vi "Server Fix.vi"() -> ()   [LabVIEW 2017]
uses:
  <vilib>/Analysis/Matrix/Datatypes/RealMatrix.ctl
  <vilib>/Platform/TimedLoop/XDataNode/timing_clust.ctl
  <vilib>/Platform/TimedLoop/XDataNode/nitl_modes.ctl
  <vilib>/Platform/TimedLoop/XDataNode/wakeup.ctl
  <vilib>/platform/TimedLoop/XDataNode/XDataNode.xnode
  <vilib>/Platform/TimedLoop/XDataNode/XDNodeRunTimeDep.lvlib
  <vilib>/Analysis/Matrix/NI_Matrix.lvlib
panel:
  in  "Processor":i32=-2
  out "?":string="SERVER"
  out "BYTE WRITE FROM SERVER":i32
  in  "Matrix":T1
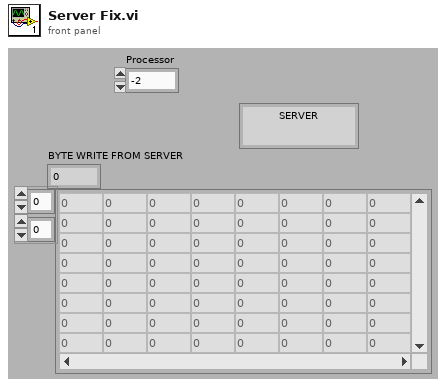
[diagram p1: front panel]
types:
  T1 = typedef "NI_Matrix.lvlib/RealMatrix.ctl" = dbl[][]
  T2 = typedef "XDNodeRunTimeDep.lvlib/timing_clust.ctl" = cluster{"Expected End [f-1]":u64, "Actual End [f-1]":u64, "Finished Late? [f-1]":bool, "Expected End [i-1]":u64, "Actual End [i-1]":u64, "Finished Late? [i-1]":bool, "Expected Start [i]":u64, "Actual Start [i]":u64, "Expected Start [f]":u64, "Actual Start [f]":u64, "Source Name":string, "Structure Name":string, "Period":i64, "Deadline":i64, "Offset":i64, "Start":i64, "Priority":i32, "Timeout":i32, "Mode":T3, "Wakeup Reason":T4, "Error":errorcluster, "Source Type":string, "Secondary Source Type":string, "Global End Time":u64, "Global Start Time":u64, "Frame Duration":u64, "Iteration Duration":u64, "Assigned CPU":i32, "I/O Scan Engine Mode":u32}
  T3 = typedef "XDNodeRunTimeDep.lvlib/nitl_modes.ctl" = enum32{"No Change", "Process missed periods, maintain original phase", "Discard missed periods, maintain original phase", "Process missed periods, ignore original phase", "Discard missed periods, ignore original phase"}
  T4 = typedef "XDNodeRunTimeDep.lvlib/wakeup.ctl" = enum32{"Normal", "Aborted", "Asynchronous wakeup", "Timing source error", "Timed loop error", "Timeout"}
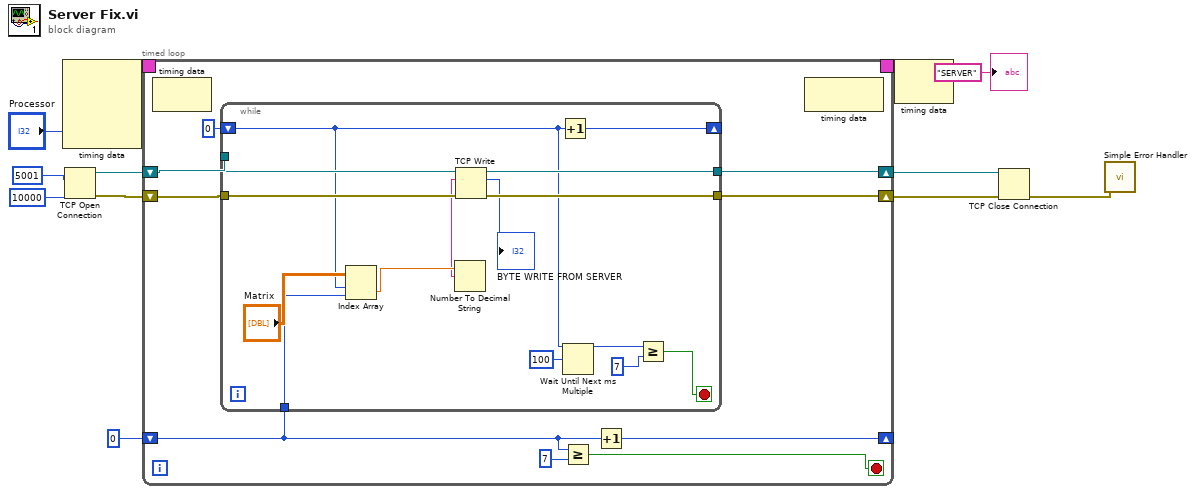
[diagram p0: block diagram]
diagram:
  n1 = node-c288("Processor") -> (w3:T2)  [unwired: 3 in]
  n2 = TCP Open Connection(remote port or service name=u16 5001, timeout ms (60000)=10000) -> (connection ID=w10:refnum<k5>, error out=w9:errorcluster)  [unwired: 3 in]
  n3 = timed-loop {
    shift-right: [w19] -> w7
    shift-left: w10 -> [w21]
    shift-right: [w18] -> w6
    shift-left: w9 -> [w20]
    shift-right: [w16] -> _
    shift-left: 0 -> [w13]
    timing: w3 -> [_]
    timing-out: [_] -> w2
    stop <- w14 stop-if-true
    n4 = node-c288() -> ()  [unwired: 1 in, 1 out]
    n5 = while {
      tunnel: w21 -> [w37]
      tunnel: w20 -> [w36]
      tunnel: [w35] -> w19
      tunnel: [w34] -> w18
      shift-right: [w28] -> _
      shift-left: 0 -> [w27]
      tunnel: w13 -> [w24]
      stop <- w25 stop-if-true
      n6 = Index Array(array="Matrix", index (row)=w27, index (col)=w24) -> (element=w31:dbl)
      n7 = Number To Decimal String(number=w31) -> (decimal integer string=w30:string)  [unwired: 1 in]
      n8 = TCP Write(connection ID=w37, data in=w30, error in (no error)=w36) -> (connection ID out=w35:refnum<k5>, bytes written=→"BYTE WRITE FROM SERVER":i32, error out=w34:errorcluster)  [unwired: 1 in]
      n9 = Increment(x=w27) -> (x+1=w28:i32)
      n10 = Wait Until Next ms Multiple(millisecond multiple=u32 100) -> ()  [unwired: 1 out]
      n11 = Greater Or Equal?(x=w27, y=7) -> (x >= y?=w25:bool)
    }
    n12 = Greater Or Equal?(x=w13, y=7) -> (x >= y?=w14:bool)
    n13 = Increment(x=w13) -> (x+1=w16:i32)
    n14 = node-c288() -> ()  [unwired: 1 in, 1 out]
  }
  n15 = node-c288(w2) -> ()  [unwired: 1 out]
  n16 = TCP Close Connection(connection ID=w7, error in (no error)=w6) -> (error out=w8:errorcluster)  [unwired: 1 in, 1 out]
  n17 = call <vilib>:"Simple Error Handler.vi"("error in (no error)"=w8) -> ()  [unwired: 4 in, 5 out]
  "?" <- "SERVER"
